vi "Periodic Tasks.vi"(8 "error in":errorcluster) -> ()   [LabVIEW 2014]
doc: "This VI runs in parallel to other tasks. It can contain as many user-defined periodic loops as you need. These can carry out PID or other sorts of timed response."
uses:
  <vilib>/Rock Robotics/WPI/Joystick/WPI_JoystickGetSetRefNum.vi
  <vilib>/Rock Robotics/WPI/RobotDrive/WPI_RobotDriveGetSetRefNum.vi
  Robot Global Data.vi
  <vilib>/Rock Robotics/WPI/Compressor/WPI_CompressorGetSetRefNum.vi
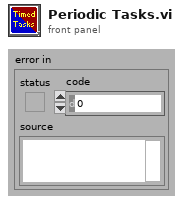
[diagram p1: front panel]
types:
  T1 = typedef "WPI_JoystickDevRef.ctl" = cluster{"Device":T2}
  T2 = typedef "WPI_JoystickDeviceEnum.ctl" = enum16{"USB 0", "USB 1", "USB 2", "USB 3", "USB 4", "USB 5"}
  T3 = typedef "WPI_RobotDriveDevRef.ctl" = cluster{"DevStatus":errorcluster, "Motors[]":T4[], "Square Inputs":bool, "Max Output":dbl}
  T4 = typedef "WPI_MotorControlDeviceRef.ctl" = cluster{"DeviceStatus":errorcluster, "Type":T5, "PWM":cluster{"Controller":T6, "PWM Channel":T7, "DeadBand":T8}, "CAN":cluster{"Device Number":u8, "Control Mode":T9, "Semaphore":T10, "Max Vout":dbl, "TalonSRX Control Mode":T11}, "Invert":bool, "TransformRef":T12, "InvTransformRef":T12}
  T5 = typedef "WPI_MotorControlType.ctl" = enum16{"PWM", "CAN", "CANTalonSRX"}
  T6 = typedef "FPGA_TypedefDigitalModule.ctl" = enum16{"Controller 1"}
  T7 = typedef "FPGA_DIOPWMChannel.ctl" = enum8{"PWM 0", "PWM 1", "PWM 2", "PWM 3", "PWM 4", "PWM 5", "PWM 6", "PWM 7", "PWM 8", "PWM 9", "PWM MXP 0", "PWM MXP 1", "PWM MXP 2", "PWM MXP 3", "PWM MXP 4", "PWM MXP 5", "PWM MXP 6", "PWM MXP 7", "PWM MXP 8", "PWM MXP 9", "Invalid"}
  T8 = typedef "WPI_PWMDeadband.ctl" = cluster{"Name":string, "maxPositivePwm":i32, "minPositivePwm":i32, "centerPwm":i32, "maxNegativePwm":i32, "minNegativePwm":i32, "angularRange":u16}
  T9 = typedef "WPI_CANJaguar_ControlMode.ctl" = enum8{"Percent VBus", "Current", "Speed", "Position", "Voltage"}
  T10 = typedef "Semaphore RefNum" = refnum<k1>
  T11 = typedef "WPI_CANTalonSRX_APIControlMode.ctl" = enum8{"Percent VBus", "Speed", "Position", "Slave", "Unchanged / Invalid"}
  T12 = typedef "WPI_PWMTransform_ConPane.ctl" = refnum<vi>
  T13 = typedef "WPI_CompressorDevRef.ctl" = cluster{"DevStatus":errorcluster, "Pneumatics Control Module":u8}
  T14 = cluster{"JoystickDevRef":T1, "RobotDriveDevRef":T3}
  T15 = cluster{"Buttons[0]":bool, "Buttons[1]":bool, "Buttons[2]":bool, "Buttons[3]":bool, "Buttons[4]":bool, "Buttons[5]":bool, "Buttons[6]":bool, "Buttons[7]":bool, "Buttons[8]":bool}
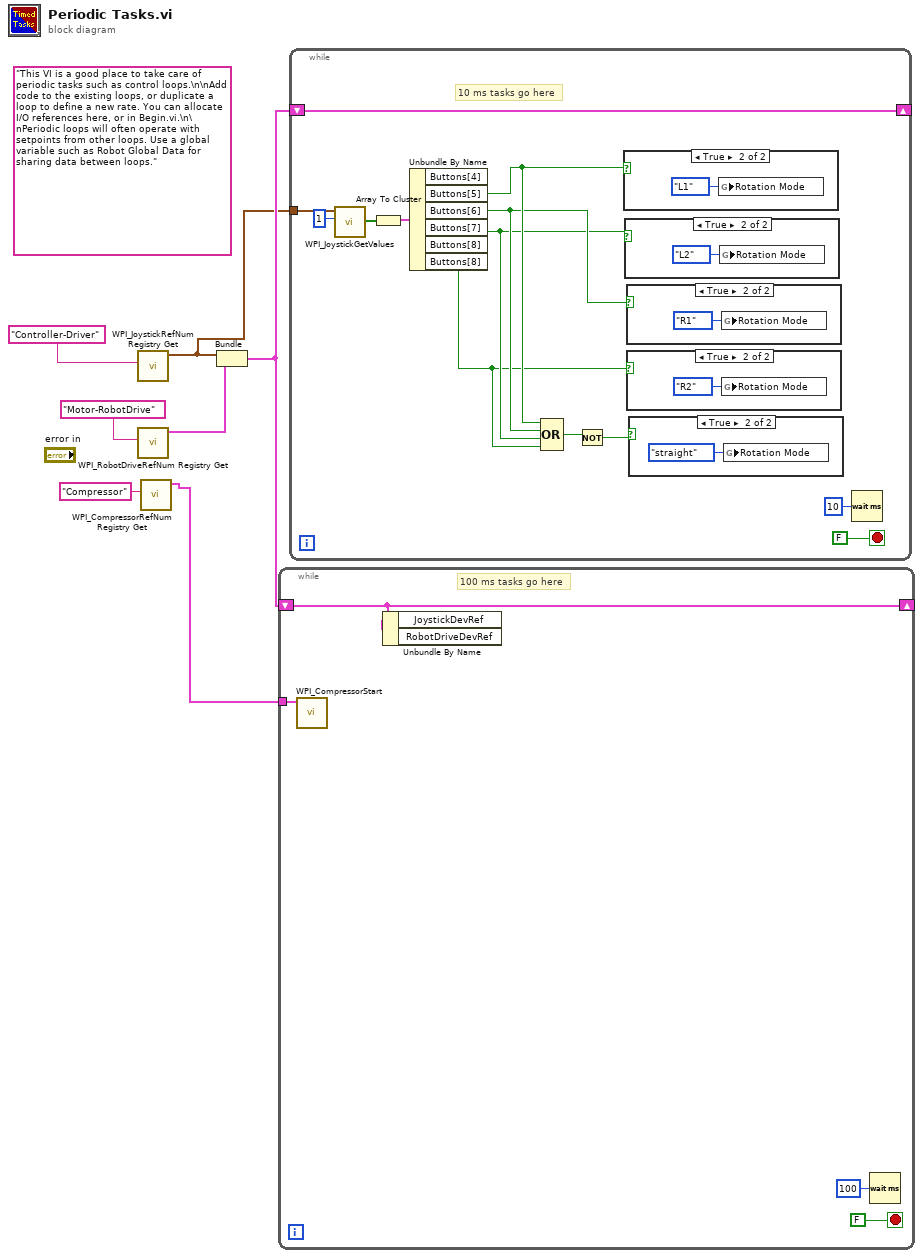
[diagram p0: block diagram]
diagram:
  (unwired) "This VI is a good place to take care of periodic tasks such as control loops.\n\nAdd code to the existing loops, or duplicate a loop to define a new rate. You can allocate I/O references here, or in Begin.vi.\n\nPeriodic loops will often operate with setpoints from other loops. Use a global variable such as Robot Global Data for sharing data between loops."
  n1 = call <vilib>:"WPI_JoystickRefNum Registry Get.vi"("refnum name"="Controller-Driver") -> ("JoystickDevRef"=w3:T1)  [unwired: 1 in, 9 out]
  n2 = call <vilib>:"WPI_RobotDriveRefNum Registry Get.vi"("refnum name"="Motor-RobotDrive") -> ("RobotDriveDevRef"=w5:T3)  [unwired: 1 in, 9 out]
  n3 = call <vilib>:"WPI_CompressorRefNum Registry Get.vi"("refnum name"="Compressor") -> ("CompressorDevRef"=w1:T13)  [unwired: 9 in, 1 out]
  n4 = Bundle("JoystickDevRef"=w3, "RobotDriveDevRef"=w5) -> (w4:T14)  [unwired: 1 out]
  n5 = while {
    shift-right: [w9] -> _
    shift-left: w4 -> [w9]
    tunnel: w1 -> [w8]
    stop <- FALSE stop-if-true
    # "100 ms tasks go here"
    n6 = call <vilib>:"WPI_CompressorStart.vi"("CompressorDevRef"=w8) -> ()  [unwired: 9 in, 2 out]
    n7 = Unbundle By Name(w9) -> ()  [unwired: 2 out]
    n8 = Wait (ms)(milliseconds to wait=u32 100) -> ()  [unwired: 1 out]
  }
  n9 = while {
    shift-right: [w22] -> _
    shift-left: w4 -> [w22]
    tunnel: w3 -> [w13]
    stop <- FALSE stop-if-true
    # "10 ms tasks go here"
    n10 = call <vilib>:"WPI_JoystickGetValues.vi"("Scaler"=i8 1, "JoystickDevRef"=w13) -> ("Buttons"=w15:bool[])  [unwired: 5 in, 4 out]
    n11 = Array To Cluster(array=w15) -> (cluster=w14:T15)
    n12 = Unbundle By Name(w14) -> ("Buttons[5]"=w21:bool, "Buttons[6]"=w20:bool, "Buttons[7]"=w19:bool, "Buttons[8]"=w18:bool)  [unwired: 2 out]
    n13 = Compound Arithmetic op=OR(w21, w20, w19, w18) -> (w17:bool)
    n14 = Not(x=w17) -> (.not. x?=w16:bool)
    n15 = case shown="True" w21 {
      frame False {
      }
      frame True {
        n16 = global write "Robot Global Data.vi" "Rotation Mode"(enum16{"straight", "L1", "L2", "R1", "R2"}."L1" ("Rotation Mode")) -> ()
      }
    }
    n17 = case shown="True" w19 {
      frame False {
      }
      frame True {
        n18 = global write "Robot Global Data.vi" "Rotation Mode"(enum16{"straight", "L1", "L2", "R1", "R2"}."L2" ("Rotation Mode")) -> ()
      }
    }
    n19 = case shown="True" w20 {
      frame False {
      }
      frame True {
        n20 = global write "Robot Global Data.vi" "Rotation Mode"(enum16{"straight", "L1", "L2", "R1", "R2"}."R1" ("Rotation Mode")) -> ()
      }
    }
    n21 = case shown="True" w18 {
      frame False {
      }
      frame True {
        n22 = global write "Robot Global Data.vi" "Rotation Mode"(enum16{"straight", "L1", "L2", "R1", "R2"}."R2" ("Rotation Mode")) -> ()
      }
    }
    n23 = case shown="True" w16 {
      frame False {
      }
      frame True {
        n24 = global write "Robot Global Data.vi" "Rotation Mode"(enum16{"straight", "L1", "L2", "R1", "R2"}."straight" ("Rotation Mode")) -> ()
      }
    }
    n25 = Wait (ms)(milliseconds to wait=u32 10) -> ()  [unwired: 1 out]
  }
